vi "Generate Report.vi"(8 "error in (no error)":errorcluster, 11 "JSON Report in":refnum<class "JSON Report.lvclass">) -> (0 "error out":errorcluster, 3 "JSON Report out":refnum<class "JSON Report.lvclass">)   [LabVIEW 2020, in "JSON Report.lvclass"]
uses:
  JSON Report.lvclass
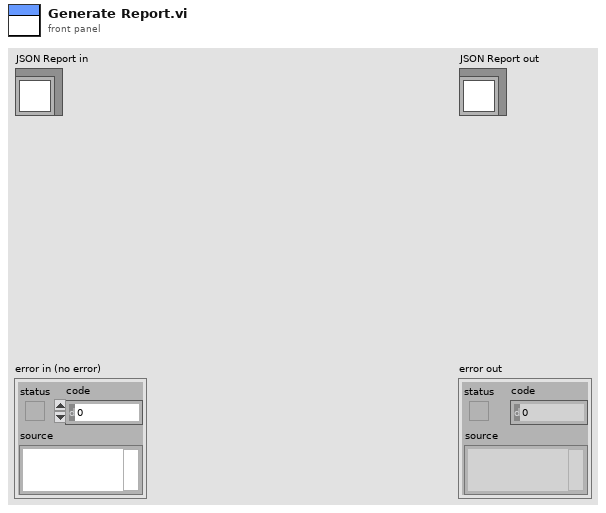
[diagram p1: front panel]
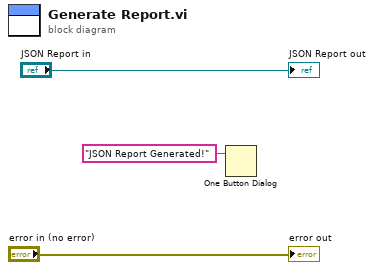
[diagram p0: block diagram]
diagram:
  n1 = One Button Dialog(message="JSON Report Generated!") -> ()  [unwired: 1 in, 1 out]
  "error out" <- "error in (no error)"
  "JSON Report out" <- "JSON Report in"
